vi "Control - Variable Geometry Turbo (VGT).vi"(8 "Control Inputs":T1={"Engine Speed [RPM]"=0.0, "Engine Status"=enum."STALLED", "Load Control \nMode"=enum."High-Idle Governor", "dt(s)"=0.0, "Number of Cylinders"=0, "Engine Displacement [cc]"=0.0, "StoichAFR"=0.0, "Q.LHV Fuel [kJ/kg]"=0.0, "BattV PSU [V]"=0.0, "12V PSU [V]"=0.0, "5V PSU [V]"=0.0, "Pedal Position [%]"=0.0, "Oil Pressure [kPa]"=0.0, "Oil Temp [C]"=0.0, "Oil Level [%]"=0.0, "Engine Coolant Temp (ECT) [C]"=0.0, "Engine Coolant Pressure [kPa]"=0.0, "Rail Pressure [bar]"=0.0, "Fuel Pressure [kPa]"=0.0, "Fuel Temp [C]"=0.0, "Vacuum Pressure [kPa]"=0.0, "Throttle Position [%]"=0.0, "Cam1 Advance [CAD]"=0.0, "Cam2 Advance [CAD]"=0.0, "Cam3 Advance [CAD]"=0.0, "Cam4 Advance [CAD]"=0.0, "CA50 Control Output [CAD]"=[], "CA50 Control Output Valid"=[], "Intake Air Temp (IAT) [C]"=0.0, "Barometric Air Pressure [kPa]"=0.0, "Intake Air Rel. Humidity [%]"=0.0, "Mass Air Flow (MAF) [kg/hr]"=0.0, "Turbo Inlet Air Pressure [kPa]"=0.0, "Turbo Inlet Air Temp [C]"=0.0, "Turbo Outlet Air Pressure [kPa]"=0.0, "Turbo Outlet Air Temp [C]"=0.0, "CAC Outlet Pressure [kPa]"=0.0, "CAC Outlet Temp [C]"=0.0, "Intake Manifold Pressure (MAP) [kPa]"=0.0, "Intake Manifold Temp (MAT) [C]"=0.0, "Exhaust Manifold Pressure [kPa]"=0.0, "Exhaust Manifold Temp [C]"=0.0, "HighP EGR Cooler Outlet Pressure [kPa]"=0.0, "HighP EGR Cooler Outlet Temp [C]"=0.0, "HighP EGR Differential Pressure [kPa]"=0.0, "HighP EGR Valve Position [%]"=0.0, "Turbo Outlet Exhaust Pressure [kPa]"=0.0, "Turbo Outlet Exhaust Temp [C]"=0.0, "VGT Position 1 [%]"=0.0, "VGT Position 2 [%]"=0.0, "Turbo Speed 1 [RPM]"=0.0, "Turbo Speed 2 [RPM]"=0.0, "LowP EGR Differential Pressure [kPa]"=0.0, "LowP EGR Valve Position [%]"=0.0, "UEGO1Lambda"=0.0, "UEGO1_Hot"=FALSE, "UEGO2Lambda"=0.0, "UEGO2_Hot"=FALSE, "Knock Intensity"=[], "Knock"=[]} {"Knock Intensity" format="%.2f"; "CA50 Control Output [CAD]" format="%.2f"; "Exhaust Manifold Temp [C]" format="%#_6f"; "UEGO2Lambda" format="%.2f"; "Intake Manifold Temp (MAT) [C]" format="%#_6f"; "UEGO1Lambda" format="%.2f"}, 11 "Intake MAP Desired [kPa]":sgl) -> (3 "VGT Position [%Open]":sgl)   [LabVIEW 2015, in "ECS-RT.lvlib"]
uses:
  ECS-RT.lvlib
  Typedefs/Control Inputs/Control Inputs.ctl
  Typedefs/EPT/Engine Status.ctl
  Typedefs/MISC/Load Control Mode.ctl
  ECS-Shared.lvlib
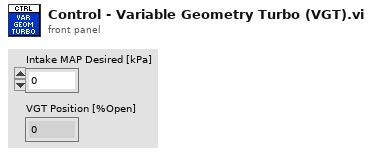
[diagram p1: front panel]
types:
  T1 = typedef "ECS-Shared.lvlib/Control Inputs.ctl" = cluster{"Engine Speed [RPM]":sgl, "Engine Status":T2, "Load Control \nMode":T3, "dt(s)":sgl, "Number of Cylinders":u8, "Engine Displacement [cc]":sgl, "StoichAFR":sgl, "Q.LHV Fuel [kJ/kg]":sgl, "BattV PSU [V]":sgl, "12V PSU [V]":sgl, "5V PSU [V]":sgl, "Pedal Position [%]":sgl, "Oil Pressure [kPa]":sgl, "Oil Temp [C]":sgl, "Oil Level [%]":sgl, "Engine Coolant Temp (ECT) [C]":sgl, "Engine Coolant Pressure [kPa]":sgl, "Rail Pressure [bar]":sgl, "Fuel Pressure [kPa]":sgl, "Fuel Temp [C]":sgl, "Vacuum Pressure [kPa]":sgl, "Throttle Position [%]":sgl, "Cam1 Advance [CAD]":sgl, "Cam2 Advance [CAD]":sgl, "Cam3 Advance [CAD]":sgl, "Cam4 Advance [CAD]":sgl, "CA50 Control Output [CAD]":sgl[], "CA50 Control Output Valid":bool[], "Intake Air Temp (IAT) [C]":sgl, "Barometric Air Pressure [kPa]":sgl, "Intake Air Rel. Humidity [%]":sgl, "Mass Air Flow (MAF) [kg/hr]":sgl, "Turbo Inlet Air Pressure [kPa]":sgl, "Turbo Inlet Air Temp [C]":sgl, "Turbo Outlet Air Pressure [kPa]":sgl, "Turbo Outlet Air Temp [C]":sgl, "CAC Outlet Pressure [kPa]":sgl, "CAC Outlet Temp [C]":sgl, "Intake Manifold Pressure (MAP) [kPa]":sgl, "Intake Manifold Temp (MAT) [C]":sgl, "Exhaust Manifold Pressure [kPa]":sgl, "Exhaust Manifold Temp [C]":sgl, "HighP EGR Cooler Outlet Pressure [kPa]":sgl, "HighP EGR Cooler Outlet Temp [C]":sgl, "HighP EGR Differential Pressure [kPa]":sgl, "HighP EGR Valve Position [%]":sgl, "Turbo Outlet Exhaust Pressure [kPa]":sgl, "Turbo Outlet Exhaust Temp [C]":sgl, "VGT Position 1 [%]":sgl, "VGT Position 2 [%]":sgl, "Turbo Speed 1 [RPM]":sgl, "Turbo Speed 2 [RPM]":sgl, "LowP EGR Differential Pressure [kPa]":sgl, "LowP EGR Valve Position [%]":sgl, "UEGO1Lambda":sgl, "UEGO1_Hot":bool, "UEGO2Lambda":sgl, "UEGO2_Hot":bool, "Knock Intensity":sgl[], "Knock":bool[]}
  T2 = typedef "ECS-Shared.lvlib/Engine Status.ctl" = enum16{"OFF", "STALLED", "CRANKING", "RUNNING", "ACCEL", "DECEL", "SAFE"}
  T3 = typedef "ECS-Shared.lvlib/Load Control Mode.ctl" = enum16{"No Governor", "Low-Idle Governor", "High-Idle Governor"}
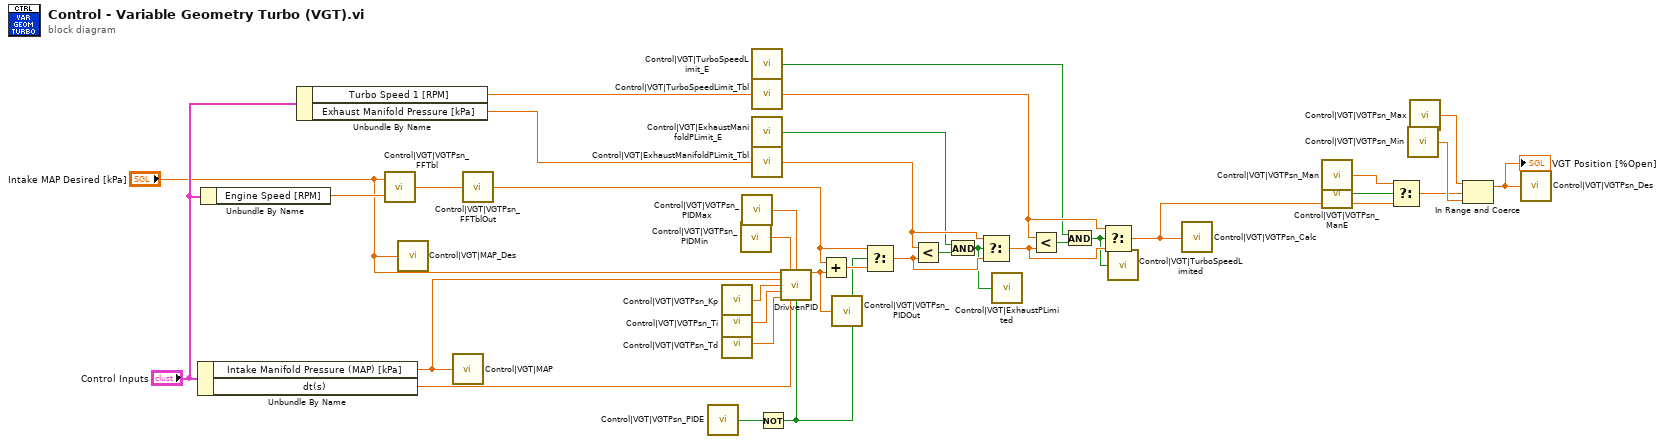
[diagram p0: block diagram]
diagram:
  n1 = Unbundle By Name("Control Inputs") -> ("Intake Manifold Pressure (MAP) [kPa]"=w1:sgl, "dt(s)"=w26:sgl)
  n2 = Unbundle By Name("Control Inputs") -> ("Engine Speed [RPM]"=w23:sgl)
  n3 = Unbundle By Name("Control Inputs") -> ("Turbo Speed 1 [RPM]"=w19:sgl, "Exhaust Manifold Pressure [kPa]"=w20:sgl)
  n4 = call "Control|VGT|VGTPsn_FFTbl"("Y Index"=w23, "X Index"="Intake MAP Desired [kPa]") -> ("Z"=w10:sgl)
  n5 = call "Control|VGT|MAP_Des"("Value"="Intake MAP Desired [kPa]") -> ()
  n6 = call "Control|VGT|MAP"("Value"=w1) -> ()
  n7 = call "Control|VGT|VGTPsn_FFTblOut"("Value"=w10) -> ()
  n8 = call "Control|VGT|VGTPsn_PIDE"() -> ("Value"=w32:bool)
  n9 = call "Control|VGT|VGTPsn_Kp"() -> ("Value"=w29:sgl)
  n10 = call "Control|VGT|VGTPsn_Ti"() -> ("Value"=w30:sgl)
  n11 = call "Control|VGT|VGTPsn_Td"() -> ("Value"=w31:sgl)
  n12 = call "Control|VGT|VGTPsn_PIDMin"() -> ("Value"=w34:sgl)
  n13 = call "Control|VGT|VGTPsn_PIDMax"() -> ("Value"=w33:sgl)
  n14 = call "Control|VGT|TurboSpeedLimit_E"() -> ("Value"=w11:bool)
  n15 = call "Control|VGT|TurboSpeedLimit_Tbl"("X Index"=w19) -> ("Y"=w16:sgl)
  n16 = call "Control|VGT|ExhaustManifoldPLimit_E"() -> ("Value"=w12:bool)
  n17 = call "Control|VGT|ExhaustManifoldPLimit_Tbl"("X Index"=w20) -> ("Y"=w17:sgl)
  n18 = Not(x=w32) -> (.not. x?=w21:bool)
  n19 = call <vilib>:"DrivvenPID.vi"("Setpoint"="Intake MAP Desired [kPa]", "OutputLow"=w34, "OutputHigh"=w33, "ProcessVariable"=w1, "ProportionalGain (Kc)"=w29, "IntegralTime (Ti, min)"=w30, "DerivativeTime (Td, min)"=w31, "dt (s)"=w26, "Reinitialize? (F)"=w21) -> ("Output"=w3:sgl)  [unwired: 6 out]
  n20 = Add(x=w10, y=w3) -> (x+y=w22:sgl)
  n21 = call "Control|VGT|VGTPsn_PIDOut"("Value"=w3) -> ()
  n22 = Select(t=w10, s=w21, f=w22) -> (s? t:f=w18:sgl)
  n23 = Less?(x=w17, y=w18) -> (x < y?=w14:bool)
  n24 = And(x=w12, y=w14) -> (x .and. y?=w6:bool)
  n25 = Select(t=w17, s=w6, f=w18) -> (s? t:f=w15:sgl)
  n26 = call "Control|VGT|ExhaustPLimited"("Value"=w6) -> ()
  n27 = Less?(x=w16, y=w15) -> (x < y?=w13:bool)
  n28 = And(x=w11, y=w13) -> (x .and. y?=w5:bool)
  n29 = Select(t=w16, s=w5, f=w15) -> (s? t:f=w9:sgl)
  n30 = call "Control|VGT|TurboSpeedLimited"("Value"=w5) -> ()
  n31 = call "Control|VGT|VGTPsn_Calc"("Value"=w9) -> ()
  n32 = call "Control|VGT|VGTPsn_Man"() -> ("Value"=w28:sgl)
  n33 = call "Control|VGT|VGTPsn_ManE"() -> ("Value"=w27:bool)
  n34 = Select(t=w28, s=w27, f=w9) -> (s? t:f=w8:sgl)
  n35 = call "Control|VGT|VGTPsn_Min"() -> ("Value"=w24:sgl)
  n36 = call "Control|VGT|VGTPsn_Max"() -> ("Value"=w25:sgl)
  n37 = In Range and Coerce(upper limit=w25, x=w8, lower limit=w24) -> (coerced(x)=w7:sgl)  [unwired: 1 out]
  "VGT Position [%Open]" <- w7
  n38 = call "Control|VGT|VGTPsn_Des"("Value"=w7) -> ()
